vi "Data Parsing.vi"(8 "error in":errorcluster, 10 "Data Read":string, 11 "Serial in":refnum<class "Serial.lvclass">) -> (0 "error out":errorcluster, 1 "Graph Data":T1, 2 "Data Out":string[](array[string]), 3 "Serial out":refnum<class "Serial.lvclass">)   [LabVIEW 2021, in "Serial.lvclass"]
uses:
  Serial.lvclass
  controls/Data for Graph.ctl
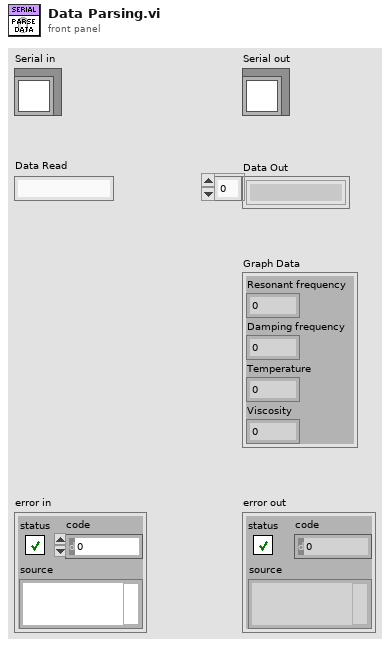
[diagram p1: front panel]
types:
  T1 = typedef "Data for Graph.ctl" = cluster{"Resonant frequency":dbl, "Damping frequency":dbl, "Temperature":dbl, "Viscosity":dbl}
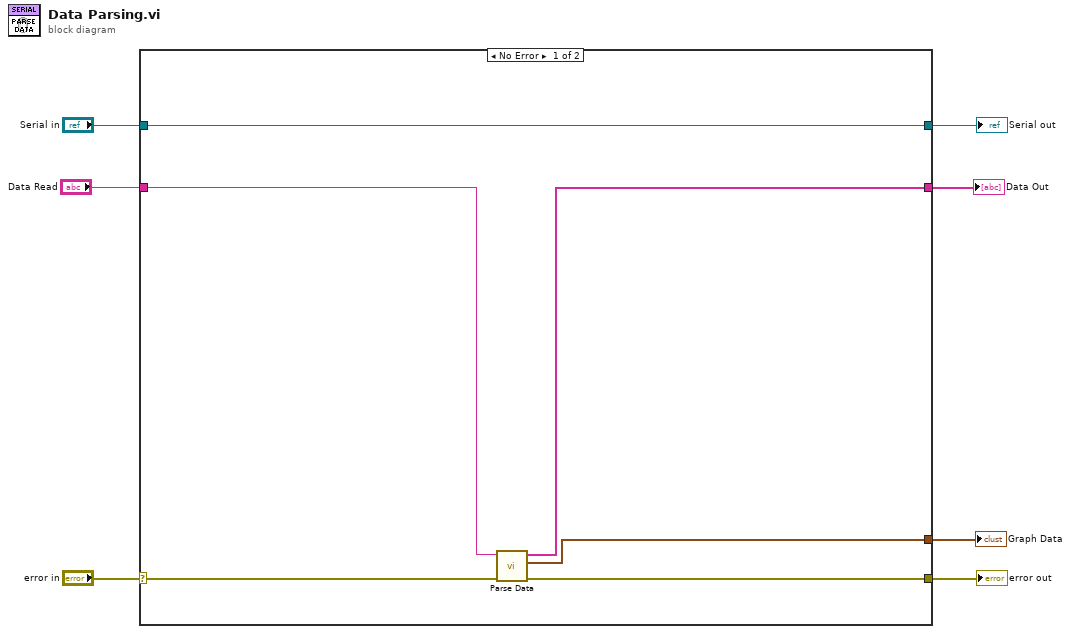
[diagram p0: block diagram]
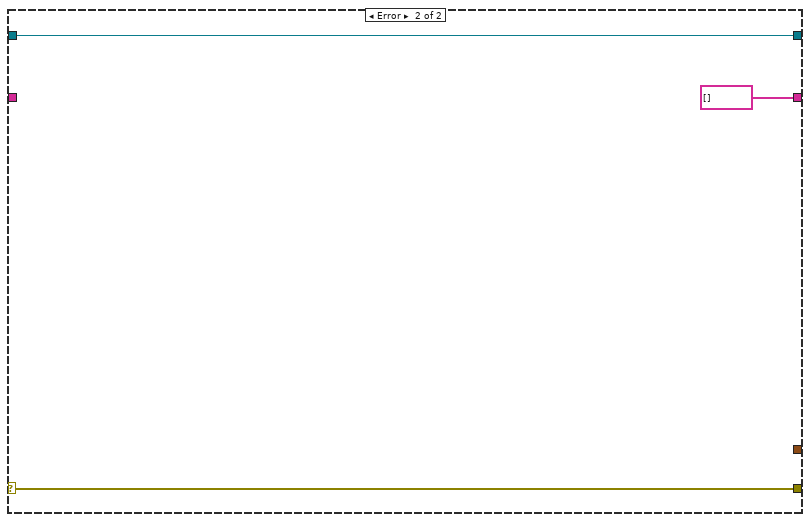
[diagram p2: hidden frame]
diagram:
  n1 = case shown="No Error" "error in" {
    selector: "error in" -> [w12 w15]
    tunnel: [w11 w15] -> w6
    tunnel: "Serial in" -> [w13 w16]
    tunnel: [w13 w16] -> w4
    tunnel: "Data Read" -> [w10 _]
    tunnel: [w9 string[] [] ("Data Out")] -> w2
    tunnel: [w8 _] -> w1
    frame No Error {
      n2 = call "Parse Data.vi"("error in"=w12, "Data Read"=w10) -> ("error out"=w11:errorcluster, "Graph Data out"=w8:T1, "Data Out"=w9:string[])  [unwired: 7 in]
    }
    frame Error {
    }
  }
  "error out" <- w6
  "Serial out" <- w4
  "Data Out" <- w2
  "Graph Data" <- w1
